vi "VI-Register XControl Events Dialog.vi"   [LabVIEW 2015]
panel:
  # "Registering XControl events..."
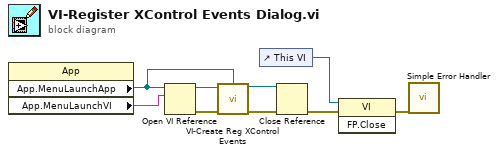
[diagram p0: block diagram]
diagram:
  n1 = property class="App"() -> ("App.MenuLaunchApp"=w1:refnum<vi>, "App.MenuLaunchVI"=w6:string)  [unwired: 2 in, 2 out]
  n2 = Open VI Reference(application reference (local)=w1, vi path=w6) -> (vi reference=w3:refnum<vi>, error out=w5:errorcluster)  [unwired: 4 in]
  n3 = call "VI-Create Reg XControl Events.vi"("VI ref in"=w3, "application refnum"=w1, "error in (no error)"=w5) -> ("VI ref out"=w2:refnum<vi>, "error out"=w4:errorcluster)  [unwired: 11 in]
  n4 = control-ref of="This VI"() -> (w7:refnum<vi>)
  n5 = Close Reference(reference=w2, error in (no error)=w4) -> (error out=w8:errorcluster)
  n6 = invoke class="VI" method="FP.Close"(reference=w7, error in=w8) -> (error out=w9:errorcluster)  [unwired: 1 in, 2 out]
  n7 = call <vilib>:"Simple Error Handler.vi"("error in (no error)"=w9) -> ()  [unwired: 4 in, 5 out]
